vi "Day07-02_녹음기.vi"() -> ()   [LabVIEW 2021]
uses:
  <vilib>/DAQmx/read.llb/DAQmx Read (Analog Wfm 1Chan NSamp).vi
  <vilib>/DAQmx/write.llb/DAQmx Write (Analog Wfm 1Chan NSamp).vi
  <vilib>/DAQmx/create/channels.llb/DAQmx Create Channel (AI-Voltage-Basic).vi
  <vilib>/DAQmx/configure/timing.llb/DAQmx Timing (Sample Clock).vi
  <vilib>/DAQmx/miscellaneous.llb/DAQmx Fill In Error Info.vi
  <vilib>/DAQmx/create/channels.llb/DAQmx Create Channel (AO-Voltage-Basic).vi
  <vilib>/DAQmx/configure/timing.llb/DAQmx Timing (Use Waveform).vi
panel:
  out "녹음기":waveform(dbl)(graph)
  in  "녹음 정지":bool
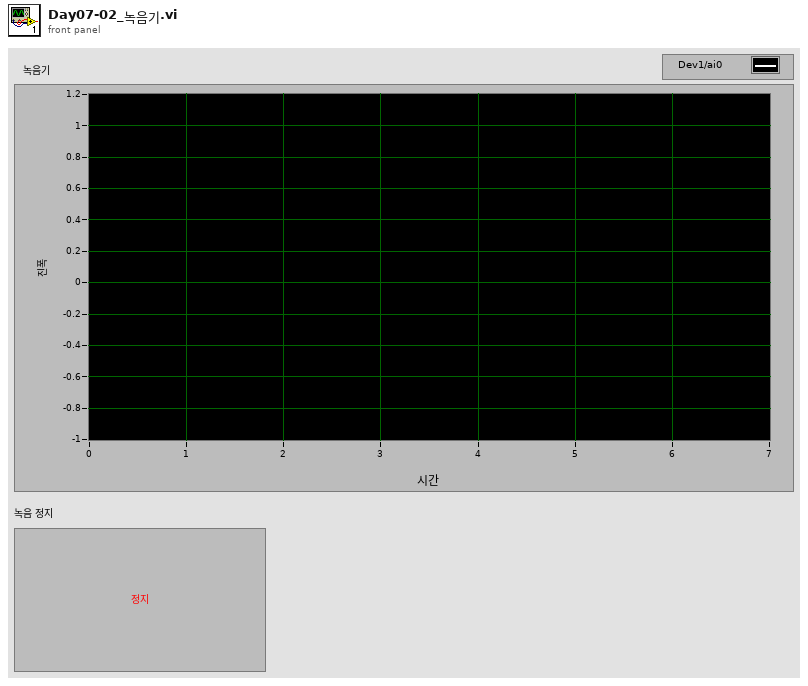
[diagram p1: front panel]
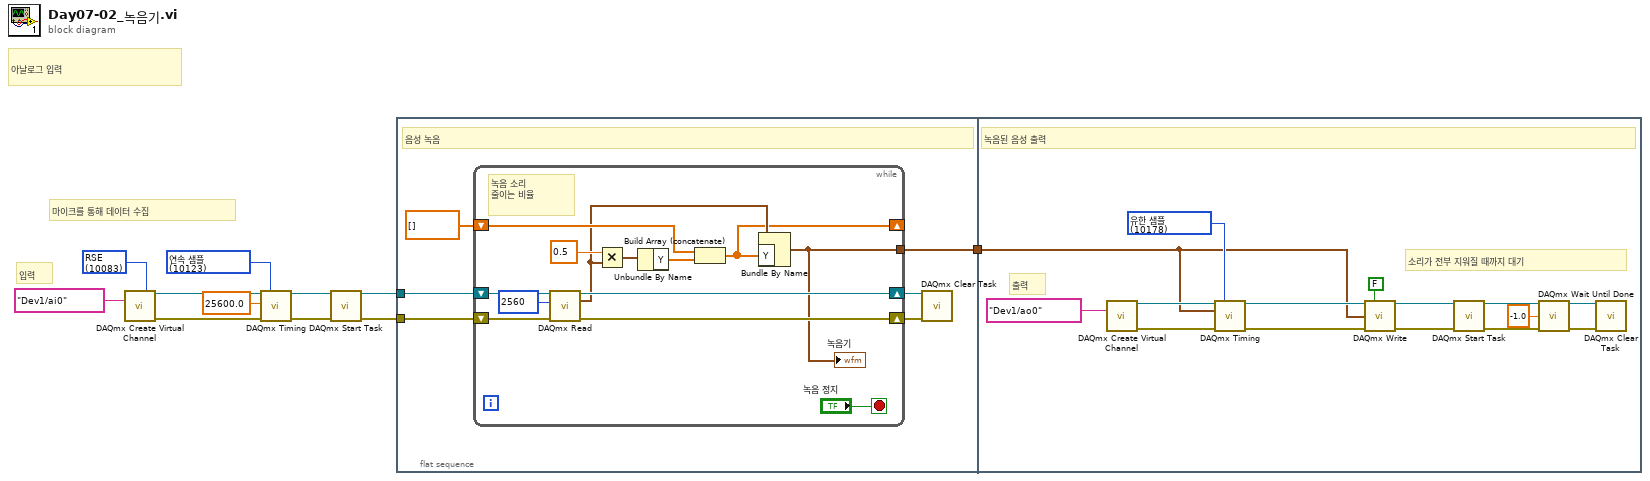
[diagram p0: block diagram]
diagram:
  w2 = 10123 items=["유한 샘플"=10178, "연속 샘플"=10123, "하드웨어 타이밍에 의한 단일 포인트"=12522] ("sample mode")
  w5 = 10083 items=["기본"=-1, "RSE"=10083, "NRSE"=10078, "차동"=10106, "유사 차동"=12529] ("input terminal configuration")
  # "마이크를 통해 데이터 수집"
  # "입력"
  # "아날로그 입력"
  n1 = call-poly <vilib>:"DAQmx Create Virtual Channel.vi"("input terminal configuration"=w5, "physical channels"=tag "Dev1/ai0") -> ("task out"=w11:refnum<k21>, "error out"=w10:errorcluster)  [unwired: 12 in]
  n2 = call-poly <vilib>:"DAQmx Timing.vi"("task/channels in"=w11, "sample mode"=w2, "rate"=25600.0, "error in"=w10) -> ("task out"=w9:refnum<k21>, "error out"=w8:errorcluster)  [unwired: 10 in]
  n3 = call <vilib>:"DAQmx Start Task.vi"("task/channels in"=w9, "error in"=w8) -> ("task out"=w7:refnum<k21>, "error out"=w6:errorcluster)  [unwired: 12 in]
  n4 = flat-sequence {
    tunnel: w7 -> [w17]
    tunnel: w6 -> [w16]
    tunnel: [w12] -> w1
    tunnel: w1 -> [w32]
    frame #0 {
      # "음성 녹음"
      n5 = while {
        shift-right: [w28] -> w15
        shift-left: w17 -> [w30]
        shift-right: [w27] -> w14
        shift-left: w16 -> [w29]
        shift-right: [w19] -> _
        shift-left: dbl[] [] -> [w21]
        tunnel: [w18] -> w12
        stop <- "녹음 정지" stop-if-true
        # "녹음 소리\n줄이는 비율"
        n6 = call-poly <vilib>:"DAQmx Read.vi"("task/channels in"=w30, "number of samples per channel"=2560, "error in"=w29) -> ("task out"=w28:refnum<k21>, "data"=w20:waveform(dbl), "error out"=w27:errorcluster)  [unwired: 10 in]
        n7 = Multiply(x=0.5, y=w20) -> (x*y=w23:waveform(dbl))
        n8 = Unbundle By Name(w23) -> ("Y"=w22:dbl[])
        n9 = Build Array (concatenate)(w21, w22) -> (w19:dbl[])
        n10 = Bundle By Name(cluster=w20, "Y"=w19) -> (w18:waveform(dbl))
        "녹음기" <- w18
      }
      n11 = call <vilib>:"DAQmx Clear Task.vi"("task in"=w15, "error in"=w14) -> ()  [unwired: 13 in, 1 out]
    }
    frame #1 {
      w33 = 10178 items=["유한 샘플"=10178, "연속 샘플"=10123, "하드웨어 타이밍에 의한 단일 포인트"=12522] ("sample mode")
      # "소리가 전부 지워질 때까지 대기"
      # "출력"
      # "녹음된 음성 출력"
      n12 = call-poly <vilib>:"DAQmx Create Virtual Channel.vi"("physical channels"=tag "Dev1/ao0") -> ("task out"=w36:refnum<k21>, "error out"=w37:errorcluster)  [unwired: 13 in]
      n13 = call-poly <vilib>:"DAQmx Timing.vi"("task/channels in"=w36, "sample mode"=w33, "waveform"=w32, "error in"=w37) -> ("task out"=w38:refnum<k21>, "error out"=w39:errorcluster)  [unwired: 10 in]
      n14 = call-poly <vilib>:"DAQmx Write.vi"("task/channels in"=w38, "auto start"=FALSE, "data"=w32, "error in"=w39) -> ("task out"=w40:refnum<k21>, "error out"=w41:errorcluster)  [unwired: 9 in, 1 out]
      n15 = call <vilib>:"DAQmx Start Task.vi"("task/channels in"=w40, "error in"=w41) -> ("task out"=w42:refnum<k21>, "error out"=w43:errorcluster)  [unwired: 12 in]
      n16 = call <vilib>:"DAQmx Wait Until Done.vi"("task/channels in"=w42, "timeout (sec)"=-1.0, "error in"=w43) -> ("task out"=w44:refnum<k21>, "error out"=w45:errorcluster)  [unwired: 11 in]
      n17 = call <vilib>:"DAQmx Clear Task.vi"("task in"=w44, "error in"=w45) -> ()  [unwired: 13 in, 1 out]
    }
  }
